vi "Read(LIST)(ALL).vi"(8 "error in":errorcluster, 11 "VISA resource name":refnum<visa-resource-name>) -> (0 "error out":errorcluster, 2 "Result":string, 3 "VISA resource name out":refnum<visa-resource-name>)   [LabVIEW 2021, in "LCR Meter.lvlib"]
doc: "Query the latest LIST measurement data of the primary parameters, secondary parameters and comparator results into the output buffer.\n\n<B>Note</B>\nOnly applicable when in the [LIST MEAS] page view."
uses:
  LCR Meter.lvlib
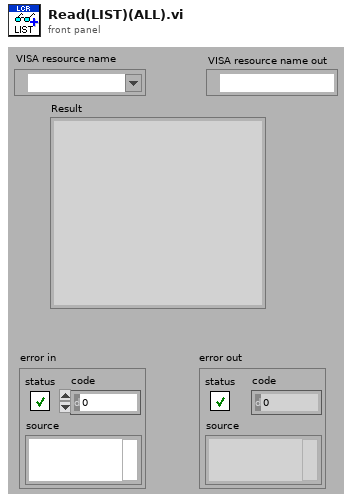
[diagram p1: front panel]
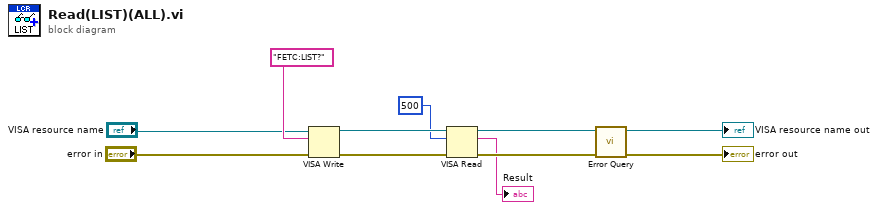
[diagram p0: block diagram]
diagram:
  n1 = VISA Write(VISA resource name="VISA resource name", write buffer="FETC:LIST?", error in (no error)="error in") -> (VISA resource name out=w11:refnum<visa-resource-name>, error out=w10:errorcluster)  [unwired: 1 out]
  n2 = VISA Read(VISA resource name=w11, byte count=u32 500, error in (no error)=w10) -> (VISA resource name out=w9:refnum<visa-resource-name>, read buffer=→"Result":string, error out=w8:errorcluster)  [unwired: 1 out]
  n3 = call "Error Query.vi"("error in (no error)"=w8, "VISA resource name"=w9) -> ("error out"=→"error out":errorcluster, "VISA resource name out"=→"VISA resource name out":refnum<visa-resource-name>)  [unwired: 6 in, 2 out]
